vi "setData.vi"(8 "error in (no error)":errorcluster, 9 "Value":i32, 10 "Tag":string, 11 "Axis in":refnum<class "Axis.lvclass">) -> (0 "error out":errorcluster, 3 "Axis out":refnum<class "Axis.lvclass">)   [LabVIEW 2019, in "Axis.lvclass"]
uses:
  Axis.lvclass
  Axis.lvclass/Axis.ctl
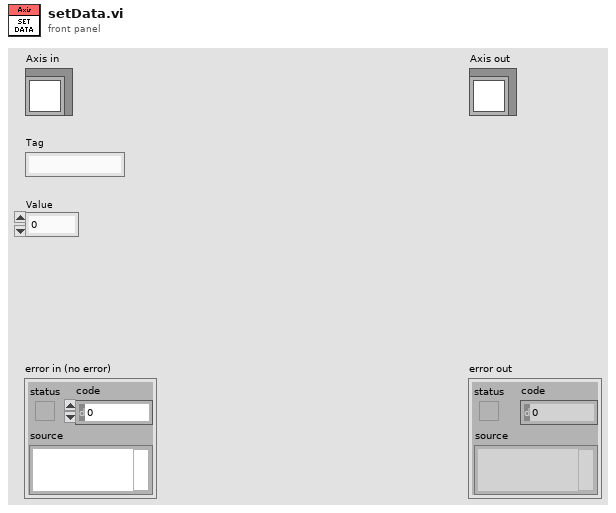
[diagram p1: front panel]
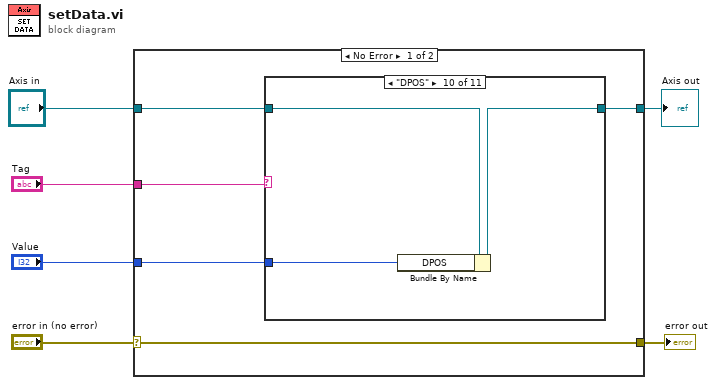
[diagram p0: block diagram]
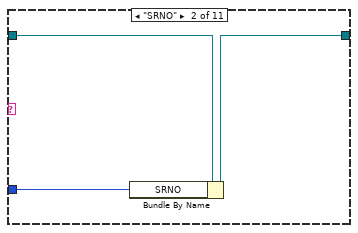
[diagram p3: hidden frame]
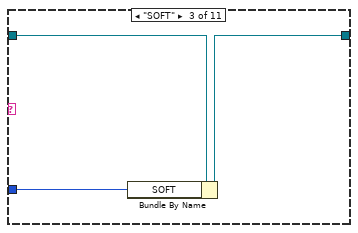
[diagram p4: hidden frame]
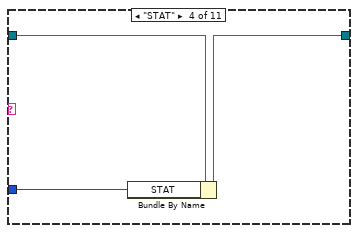
[diagram p5: hidden frame]
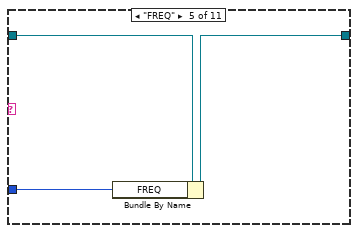
[diagram p6: hidden frame]
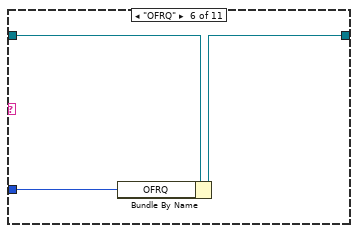
[diagram p7: hidden frame]
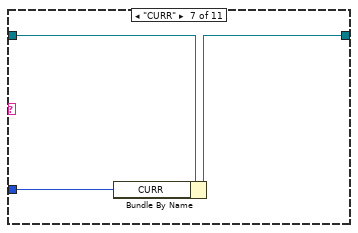
[diagram p8: hidden frame]
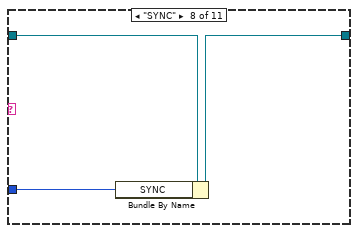
[diagram p9: hidden frame]
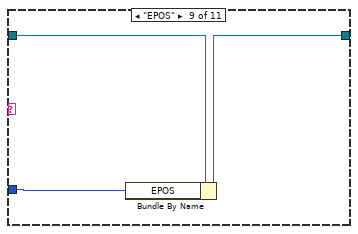
[diagram p10: hidden frame]
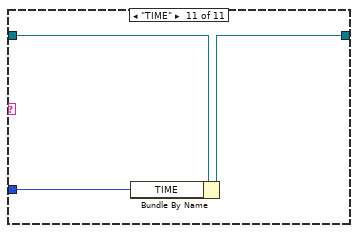
[diagram p11: hidden frame]
diagram:
  n1 = case shown="No Error" "error in (no error)" {
    selector: "error in (no error)" -> [w11 w44]
    tunnel: [w11 w44] -> w5
    tunnel: [w10 w43] -> w3
    tunnel: "Axis in" -> [w9 w43]
    tunnel: "Value" -> [w8 _]
    tunnel: "Tag" -> [w7 _]
    frame No Error {
      n2 = case shown="\"DPOS\"" w7 {
        tunnel: w9 -> [w12 w15 w16 w21 w24 w27 w30 w33 w36 w39 w42]
        tunnel: w8 -> [_ w14 w18 w20 w23 w25 w28 w32 w35 w38 w41]
        tunnel: [w12 w13 w17 w19 w22 w26 w29 w31 w34 w37 w40] -> w10
        frame Default {
        }
        frame "SRNO" {
          n3 = Bundle By Name(cluster=w15, "SRNO"=w14) -> (w13:refnum<class "Axis.lvclass">)
        }
        frame "SOFT" {
          n4 = Bundle By Name(cluster=w16, "SOFT"=w18) -> (w17:refnum<class "Axis.lvclass">)
        }
        frame "STAT" {
          n5 = Bundle By Name(cluster=w21, "STAT"=w20) -> (w19:refnum<class "Axis.lvclass">)
        }
        frame "FREQ" {
          n6 = Bundle By Name(cluster=w24, "FREQ"=w23) -> (w22:refnum<class "Axis.lvclass">)
        }
        frame "OFRQ" {
          n7 = Bundle By Name(cluster=w27, "OFRQ"=w25) -> (w26:refnum<class "Axis.lvclass">)
        }
        frame "CURR" {
          n8 = Bundle By Name(cluster=w30, "CURR"=w28) -> (w29:refnum<class "Axis.lvclass">)
        }
        frame "SYNC" {
          n9 = Bundle By Name(cluster=w33, "SYNC"=w32) -> (w31:refnum<class "Axis.lvclass">)
        }
        frame "EPOS" {
          n10 = Bundle By Name(cluster=w36, "EPOS"=w35) -> (w34:refnum<class "Axis.lvclass">)
        }
        frame "DPOS" {
          n11 = Bundle By Name(cluster=w39, "DPOS"=w38) -> (w37:refnum<class "Axis.lvclass">)
        }
        frame "TIME" {
          n12 = Bundle By Name(cluster=w42, "TIME"=w41) -> (w40:refnum<class "Axis.lvclass">)
        }
      }
    }
    frame Error {
    }
  }
  "error out" <- w5
  "Axis out" <- w3
